vi "Start Thread.vi"(8 "error in (no error)":errorcluster, 11 "Template":refnum<class "Singleton.lvclass">) -> (0 "error out":errorcluster, 3 "object":refnum<class "Singleton.lvclass">)   [LabVIEW 2014, in "Singleton.lvlib" / "Singleton.lvclass"]
uses:
  Singleton.lvclass
  Singleton.lvclass/Singleton.ctl
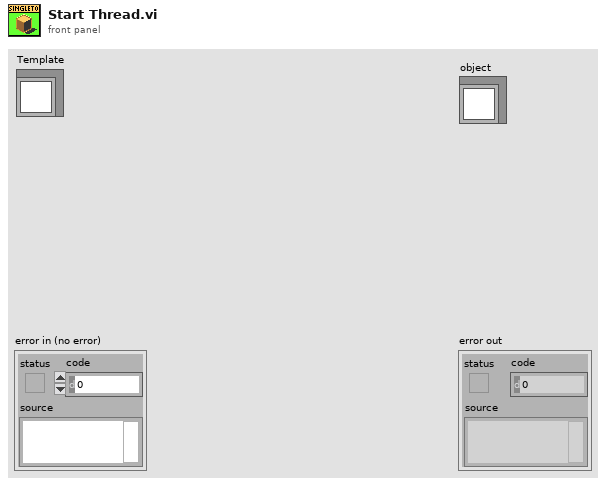
[diagram p1: front panel]
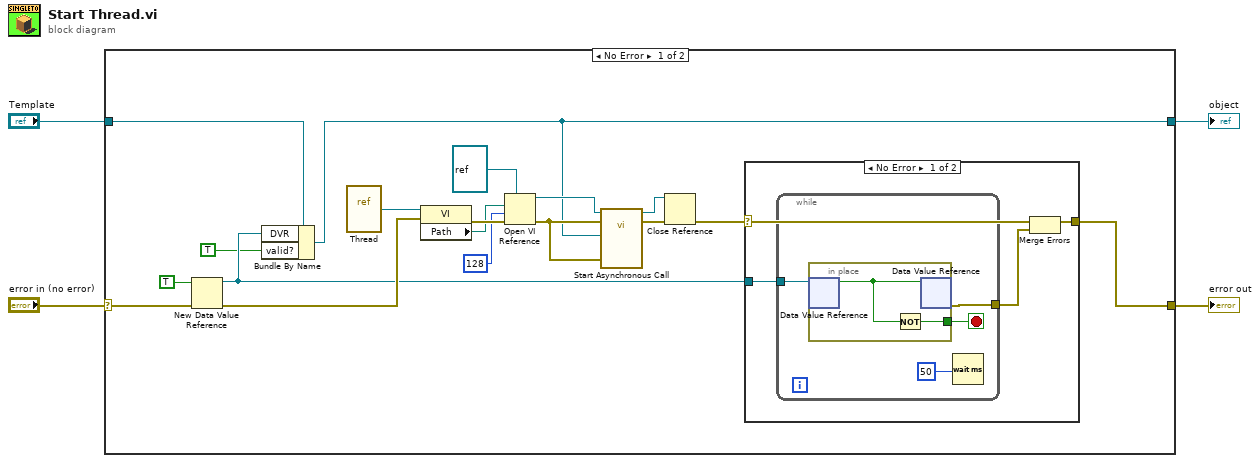
[diagram p0: block diagram]
diagram:
  n1 = case shown="No Error" "error in (no error)" {
    selector: "error in (no error)" -> [w12 w35]
    tunnel: [w9 w34] -> w3
    tunnel: "Template" -> [w10 w34]
    tunnel: [w7 w35] -> w1
    frame No Error {
      n2 = New Data Value Reference(data value=TRUE, error in=w12) -> (data value reference=w8:refnum<data-value>, error out=w11:errorcluster)
      n3 = Bundle By Name(cluster=w10, "DVR"=w8, "valid?"=TRUE) -> (w9:refnum<class "Singleton.lvclass">)
      n4 = vi-ref "Thread.vi"() -> (w22:refnum<vi>)
      n5 = property class="VI"(reference=w22, error in=w11) -> (error out=w21:errorcluster, "Path"=w20:path)  [unwired: 1 out]
      n6 = Open VI Reference(type specifier VI Refnum (for type only)=refnum<vi> refnum, vi path=w20, options=128, error in (no error)=w21) -> (vi reference=w19:refnum<vi>, error out=w15:errorcluster)  [unwired: 2 in]
      n7 = call-by-ref "Start Asynchronous Call"(reference=w19, error in=w15, 8:"error in (no error)"=w15, "Singleton in"=w9) -> (reference out=w17:refnum<vi>, error out=w18:errorcluster)  [unwired: 9 in, 1 out]
      n8 = Close Reference(reference=w17, error in (no error)=w18) -> (error out=w14:errorcluster)
      n9 = case shown="No Error" w14 {
        selector: w14 -> [w23 w33]
        tunnel: w8 -> [w26 _]
        tunnel: [w24 w33] -> w7
        frame No Error {
          n10 = while {
            tunnel: w26 -> [w30]
            tunnel: [w29] -> w25
            stop <- w28 stop-if-true
            n11 = in-place {
              in-place-border: [w32] -> w28
              n12 = in-place-dvr #1(w30) -> (w31:bool)  [unwired: 1 out]
              n13 = Not(x=w31) -> (.not. x?=w32:bool)
              n14 = in-place-dvr #1(w31) -> (w29:errorcluster)  [unwired: 1 out]
            }
            n15 = Wait (ms)(milliseconds to wait=u32 50) -> ()  [unwired: 1 out]
          }
          n16 = Merge Errors(w23, w25) -> (w24:errorcluster)
        }
        frame Error {
        }
      }
    }
    frame Error {
    }
  }
  "error out" <- w1
  "object" <- w3
